vi "Configure Jitter Spectrum Settings.vi"(0 "VISA resource name":refnum<visa-resource-name>, 5 "Window Mode (0: Hanning)":i32(ring) items=["Hanning", "Flat Top", "Rectangular"], 7 "Spectrum Horizontal":T2, 9 "Spectrum Vertical":T1, 11 "error in (no error)":errorcluster) -> (4 "VISA resource name out":refnum<visa-resource-name>, 15 "error out":errorcluster)   [LabVIEW 2009, in "Agilent 8000 Series.lvlib"]
doc: "Configures the Jitter Spectrum analysis and its parameters."
uses:
  Agilent 8000 Series.lvlib
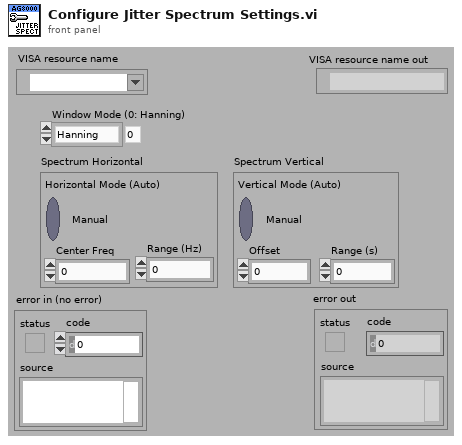
[diagram p1: front panel]
types:
  T1 = cluster{"Vertical Mode (Auto)":bool, "Offset":dbl, "Range (s)":dbl}
  T2 = cluster{"Horizontal Mode (Auto)":bool, "Center Freq":dbl, "Range (Hz) ":dbl}
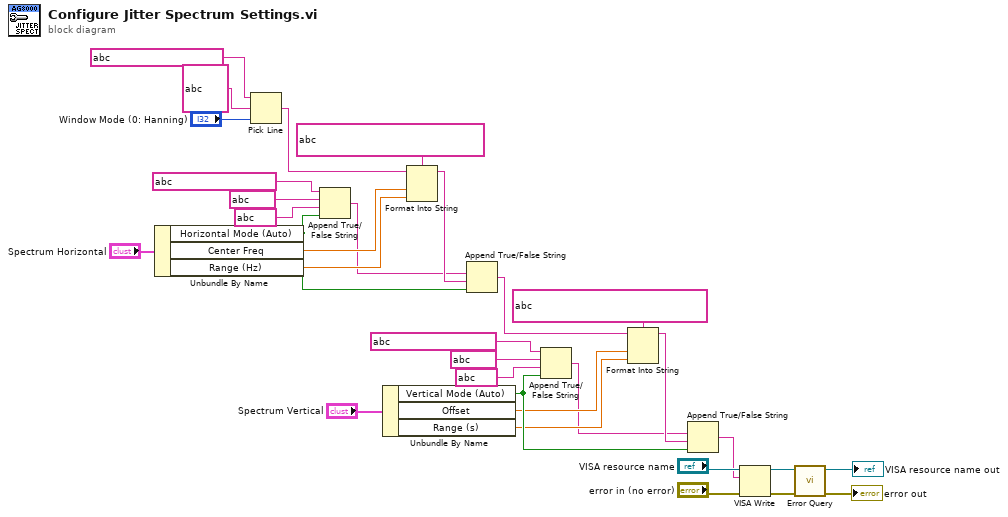
[diagram p0: block diagram]
diagram:
  n1 = Unbundle By Name("Spectrum Horizontal") -> ("Horizontal Mode (Auto)"=w14:bool, "Center Freq"=w24:dbl, "Range (Hz)"=w23:dbl)
  n2 = Pick Line(string ("")=string ?, multi-line string=string ?, line index="Window Mode (0: Hanning)") -> (output string=w1:string)
  n3 = Append True/False String(1:w14, 2:string ? ("false string"), 3:string ? ("true string"), 4:string ? ("string (\"\")")) -> (0:w15:string)
  n4 = Unbundle By Name("Spectrum Vertical") -> ("Vertical Mode (Auto)"=w13:bool, "Offset"=w7:dbl, "Range (s)"=w8:dbl)
  n5 = Format Into String(format string=string ?, initial string=w1, w24, w23) -> (resulting string=w16:string)  [unwired: 1 in, 1 out]
  n6 = Append True/False String(1:w14, 2:w16, 3:w15) -> (0:w2:string)  [unwired: 1 in]
  n7 = Append True/False String(1:w13, 2:string ? ("false string"), 3:string ? ("true string"), 4:string ? ("string (\"\")")) -> (0:w4:string)
  n8 = Format Into String(format string=string ?, initial string=w2, w7, w8) -> (resulting string=w12:string)  [unwired: 1 in, 1 out]
  n9 = Append True/False String(1:w13, 2:w12, 3:w4) -> (0:w3:string)  [unwired: 1 in]
  n10 = VISA Write(VISA resource name="VISA resource name", write buffer=w3, error in (no error)="error in (no error)") -> (VISA resource name out=w30:refnum<visa-resource-name>, error out=w29:errorcluster)  [unwired: 1 out]
  n11 = call "Error Query.vi"("error in (no error)"=w29, "VISA resource name"=w30) -> ("error out"=→"error out":errorcluster, "VISA resource name out"=→"VISA resource name out":refnum<visa-resource-name>)  [unwired: 6 in, 2 out]
